vi "SP Formulate Marker Format String.vi"(0 "X Value":dbl, 1 "Y Value":dbl) -> (6 "Format String":string)   [LabVIEW 2011]
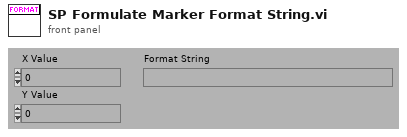
[diagram p1: front panel]
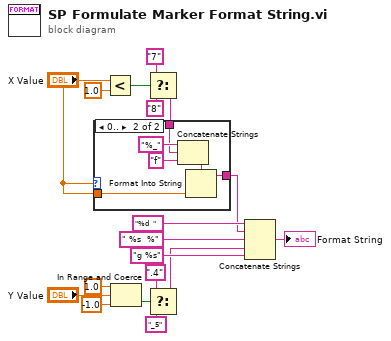
[diagram p0: block diagram]
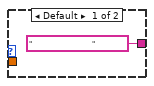
[diagram p2: hidden frame]
diagram:
  n1 = Less?(x="X Value", y=1.0) -> (x < y?=w9:bool)
  n2 = In Range and Coerce(upper limit=1.0, x="Y Value", lower limit=-1.0) -> (In Range?=w17:bool)  [unwired: 1 out]
  n3 = Select(t="7" ("format string"), s=w9, f="8" ("format string")) -> (s? t:f=w4:string)
  n4 = case shown="0.." "X Value" {
    tunnel: w4 -> [_ w23]
    tunnel: "X Value" -> [_ w21]
    tunnel: ["                              " w20] -> w2
    frame Default {
    }
    frame 0.. {
      n5 = Concatenate Strings("%_" ("format string"), w23, "f" ("format string")) -> (w22:string)
      n6 = Format Into String(format string=w22, w21) -> (resulting string=w20:string)  [unwired: 2 in, 1 out]
    }
  }
  n7 = Select(t=".4" ("format string"), s=w17, f="_5" ("format string")) -> (s? t:f=w1:string)
  n8 = Concatenate Strings("%d  " ("format string"), w2, " %s  %" ("format string"), w1, "g %s" ("format string")) -> (→"Format String":string)
